vi "Proboscis.vi"() -> ()   [LabVIEW 2017]
panel:
  out "Improved\nThreshold":T1(plugin-control)
  out "Threshold":T1(plugin-control)
  in  "Parameters":T2={"Look for"=0, "Window Size(32x32)"={"SizeX"=32, "SizeY"=32}, "Niblack Deviation Factor"=0.2, "Range"={"Lower value"=128, "Upper value"=255}, "Number of Erosion"=2} {"Range"."Upper value" scale=0.0..255.0; "Range"."Lower value" scale=0.0..255.0; "Niblack Deviation Factor" min=0.0 max=1.0 format="%.2f"; "Window Size(32x32)"."SizeY" min=3 step=1; "Window Size(32x32)"."SizeX" min=3 step=1; "Look for" items=["Bright Objects", "Dark Objects"]}
  in  "Method":i32(ring) items=["Niblack", "Background Correction", "Constant Threshold", "Auto Threshold"]
  in  "stop":bool
  in  "Frame":i32(slide) min=0 max=6 step=1 scale=0.0..6.0
  out "Original":T1(plugin-control)
  in  "JPG or AVI":bool
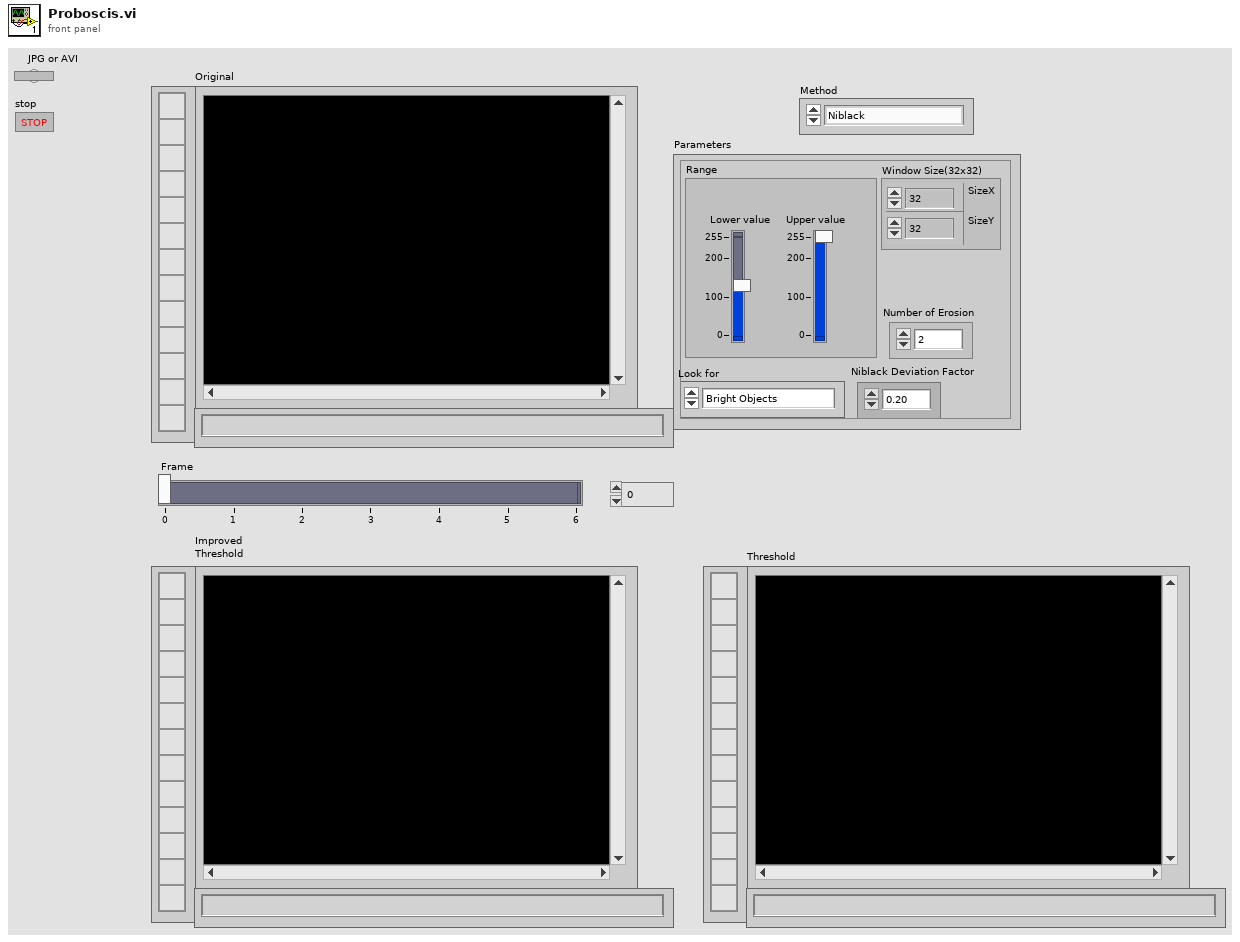
[diagram p1: front panel]
types:
  T1 = typedef "IMAQ Image.ctl" = refnum<image>
  T2 = cluster{"Look for":i32, "Window Size(32x32)":cluster{"SizeX":i32, "SizeY":i32}, "Niblack Deviation Factor":dbl, "Range":cluster{"Lower value":i32, "Upper value":i32}, "Number of Erosion":i32}
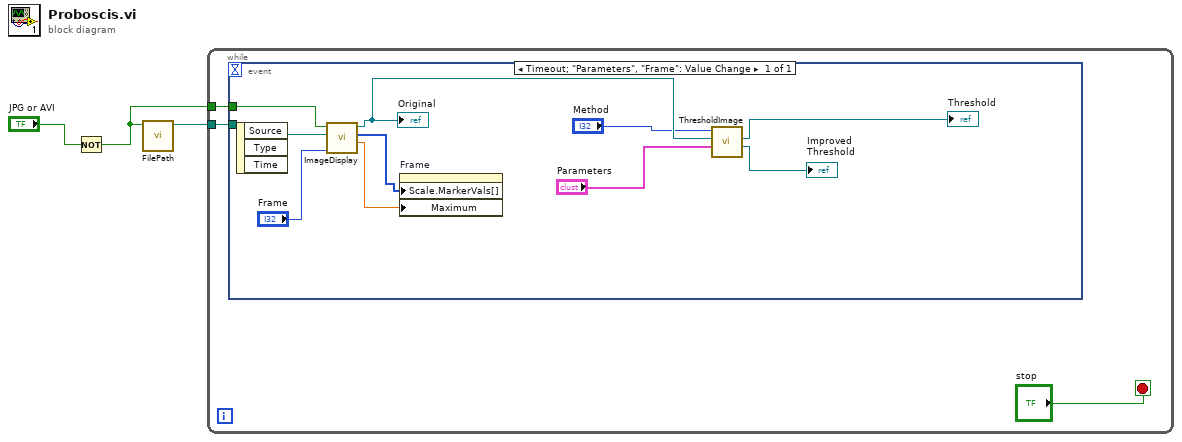
[diagram p0: block diagram]
diagram:
  n1 = Not(x="JPG or AVI") -> (.not. x?=w1:bool)
  n2 = call "FilePath.vi"("JPG or AVI"=w1) -> ("Path"=w3:path)  [unwired: 10 in]
  n3 = while {
    tunnel: w3 -> [w6]
    tunnel: w1 -> [w5]
    stop <- "stop" stop-if-true
    n4 = event shown="[0] Timeout;  \"Parameters\", \"Frame\": Value Change" {
      selector: _ -> [_]
      dyn-events: _ -> [_]
      timeout: _ -> [_]
      tunnel: w6 -> [w16]
      tunnel: w5 -> [w15]
      event Timeout; "Parameters", "Frame": Value Change {
        n5 = event-data() -> ()  [unwired: 1 in, 3 out]
        n6 = call "ImageDisplay.vi"("Frame"="Frame", "Path"=w16, "JPG or AVI"=w15) -> ("Number of frames"=w12:dbl, "Frames"=w13:u32[], "Image"=w11:T1)  [unwired: 5 in]
        "Original" <- w11
        n7 = property on="Frame" class="Slide (strict)"("Scale.MarkerVals[]"=w13, "Maximum"=w12) -> ()  [unwired: 2 in, 2 out]
        n8 = call "ThresholdImage.vi"("Method"="Method", "Image Src"=w11, "Parameters"="Parameters") -> ("Threshold"=→"Threshold":T1, "Improved Threshold"=→"Improved\nThreshold":T1)  [unwired: 6 in]
      }
    }
  }
